vi "FPGA_target_write_fifo.vi"(5 "write_FIFO":bool, 6 "mem2_addr_in":u32, 7 "mem_data_in":T1, 8 "mem2_data":u16) -> (10 "mem2_addr_dup":u32, 13 "mem_data_dup":T1, 19 "FIFO_full":bool)   [LabVIEW 2014]
doc: "writes data to internal FIFOs that used to buffer the data during pattern generation"
uses:
  FPGA_mem_data_type.ctl
  <vilib>/rvi/FIFO/Fifo_Resource/nirvififoEmulationDetermineInputValidOut.vi
  <vilib>/rvi/Emulation/niFpgaProcessEmulError.vi
  <vilib>/rvi/eio/common/nirviEmuReportErrorAndStop.vi
  <vilib>/rvi/errors/nirviReportUnexpectedCaseInternalError.vi
  <vilib>/rvi/errors/nirviReportUnexpectedCaseInternalError (U32).vi
  <vilib>/rvi/occurrence/nirviWaitOnOccurrenceBase.vi
  <vilib>/rvi/FIFO/Fifo_Resource/nirvififoEmulationReleaseLock.vi
  <vilib>/rvi/FIFO/Fifo_Resource/nirvififoEmulationObtainLock.vi
  <vilib>/rvi/FIFO/Fifo_Resource/nirvififoEmulationCreateLock.vi
  <vilib>/rvi/DataTransferAndStorage/Container/Common/niFpgaContainerGetUniqueNameForEmu.vi
  <vilib>/rvi/FIFO/Fifo_Resource/nirvififoEmulationSetSize.vi
  <vilib>/rvi/FIFO/Fifo_Resource/nirviFifoEmulationQueueMgr.vi
  <instcachedir>/0/nirviFifoEmulationQueueMgr_E5CAEC123FF24DC58D834DCA3CDAA9B5.lvgen/nirviFifoEmulationQueueMgr_E5CAEC123FF24DC58D834DCA3CDAA9B5_002.vi
  <vilib>/rvi/errors/niFpgaSetErrorForExecOnDevCompSimple.vi
  <vilib>/rvi/Emulation/niFpgaSctlEmulationGetInTimedLoop.vi
  <vilib>/rvi/Emulation/niFpgaEmulationIsFPGAContextNoSignature.vi
  <instcachedir>/0/nirviFifoEmulationQueueMgr_E5CAEC123FF24DC58D834DCA3CDAA9B5.lvgen/nirviFifoEmulationQueueMgr_E5CAEC123FF24DC58D834DCA3CDAA9B5_001.vi
  <instcachedir>/0/nirviFifoEmulationQueueMgr_E5CAEC123FF24DC58D834DCA3CDAA9B5.lvgen/nirviFifoEmulationQueueMgr_E5CAEC123FF24DC58D834DCA3CDAA9B5_003.vi
  <vilib>/rvi/Emulation/niFpgaSctlEmulationResourceMgr.vi
  <vilib>/rvi/Memory/Memory_Emulation/nirvimemoryEmulationManagerCache_SetValue.vi
  <vilib>/rvi/Memory/Memory_Emulation/nirvimemoryEmulationManagerCache_GetValue.vi
  <vilib>/rvi/Memory/Memory_Emulation/nirvimemoryEmulationManagerCache_ReleaseExclusive.vi
  <vilib>/Utility/error.llb/Clear Errors.vi
  <vilib>/rvi/Memory/Memory_Emulation/nirvimemoryEmulationManagerCache_InsertValue.vi
  <vilib>/rvi/Memory/Memory_Emulation/niFpgaMemoryEmulationValidateCache.vi
  <vilib>/rvi/Memory/Memory_Emulation/nirvimemoryEmulationManagerCache_MakeExclusive.vi
  <vilib>/rvi/Memory/Memory_Emulation/niFpgaMemoryEmulationCacheClearOnFirstRun.vi
  <vilib>/rvi/Memory/Memory_Emulation/nirvimemoryEmulation.vi
  <vilib>/rvi/Memory/Memory_Emulation/nirvimemoryFastEmulation.vi
  <vilib>/rvi/DataTransferAndStorage/Container/XNode/niFpgaContainer.xnode
  <vilib>/rvi/FIFO/Fifo_Resource/nirvififoEmulationWrite.vi
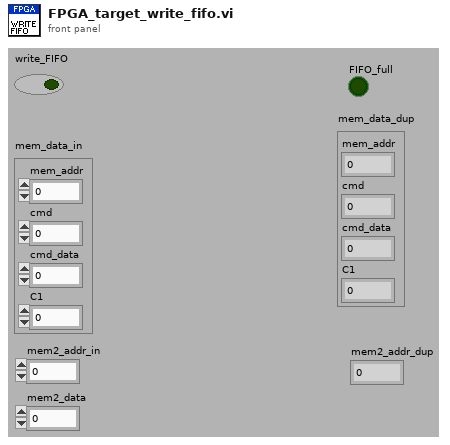
[diagram p1: front panel]
types:
  T1 = typedef "FPGA_mem_data_type.ctl" = cluster{"mem_addr":u32, "cmd":u8, "cmd_data":u32, "C1":u16}
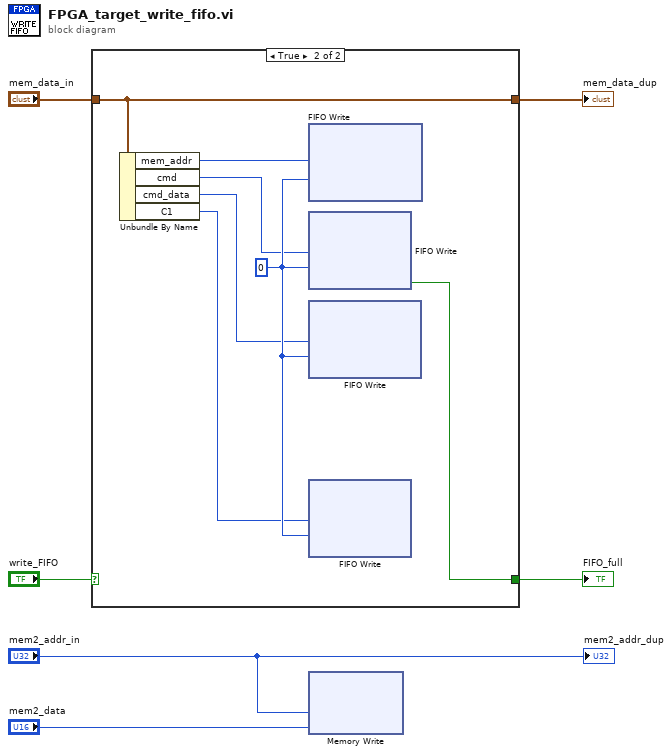
[diagram p0: block diagram]
diagram:
  n1 = case shown="True" "write_FIFO" {
    tunnel: [_ w14] -> w6
    tunnel: "mem_data_in" -> [w7 w10]
    tunnel: [w7 w10] -> w1
    frame False {
    }
    frame True {
      w13 = 0 ("Timeout")
      n2 = Unbundle By Name(w10) -> ("mem_addr"=w9:u32, "cmd"=w12:u8, "cmd_data"=w11:u32, "C1"=w8:u16)
      n3 = xnode ("FIFO Write")("Element"=w9, "Timeout"=w13) -> ()  [unwired: 1 in, 2 out]
      n4 = xnode ("FIFO Write")("Element"=w12, "Timeout"=w13) -> ("Timed Out?"=w14:bool)  [unwired: 1 in, 1 out]
      n5 = xnode ("FIFO Write")("Element"=w11, "Timeout"=w13) -> ()  [unwired: 1 in, 2 out]
      n6 = xnode ("FIFO Write")("Element"=w8, "Timeout"=w13) -> ()  [unwired: 1 in, 2 out]
    }
  }
  "FIFO_full" <- w6
  "mem_data_dup" <- w1
  n7 = xnode ("Memory Write")("Address"="mem2_addr_in", "Data"="mem2_data") -> ()  [unwired: 1 in, 1 out]
  "mem2_addr_dup" <- "mem2_addr_in"
